vi "Write Core Reader Handle.vi"(8 "error in":errorcluster, 10 "core reader handle":u64, 11 "execution unit in":refnum<class "Execution Unit.lvclass">) -> (0 "error out":errorcluster, 3 "execution unit out":refnum<class "Execution Unit.lvclass">)   [LabVIEW 2020, in "AIM MIL-STD-1553 Engine.lvlib" / "Implementation.lvlib" / "Execution Unit.lvclass"]
uses:
  Execution Unit.lvclass
  Execution Unit.lvclass/Execution Unit.ctl
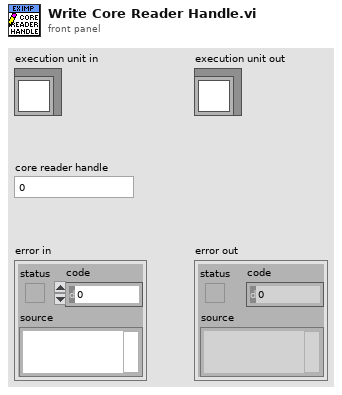
[diagram p1: front panel]
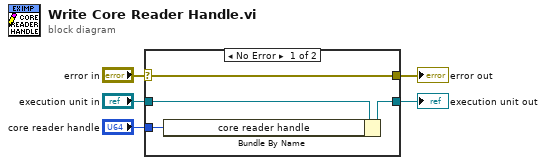
[diagram p0: block diagram]
diagram:
  n1 = case shown="No Error" "error in" {
    selector: "error in" -> [w9 w10]
    tunnel: [w9 w10] -> w4
    tunnel: [w7 w11] -> w2
    tunnel: "execution unit in" -> [w8 w11]
    tunnel: "core reader handle" -> [w6 _]
    frame No Error {
      n2 = Bundle By Name(cluster=w8, "core reader handle"=w6) -> (w7:refnum<class "Execution Unit.lvclass">)
    }
    frame Error {
    }
  }
  "error out" <- w4
  "execution unit out" <- w2
